vi "to_json.vi"(8 "error in":errorcluster, 11 "source in":refnum<class "source.lvclass">) -> (0 "error out":errorcluster, 2 "json":string, 3 "source out":refnum<class "source.lvclass">, 4 "Not Default":bool)   [LabVIEW 2020, in "datasources.lvlib" / "source.lvclass"]
uses:
  source.lvclass
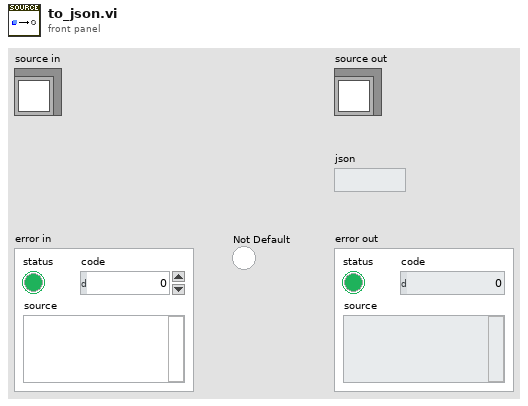
[diagram p1: front panel]
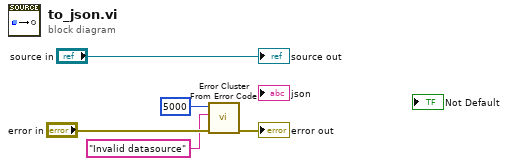
[diagram p0: block diagram]
diagram:
  n1 = call <vilib>:"Error Cluster From Error Code.vi"("error in (no error)"="error in", "error message (\"\")"="Invalid datasource" ("error message (\"\")"), "error code (0)"=5000) -> ("error out"=→"error out":errorcluster)  [unwired: 6 in]
  "source out" <- "source in"
